vi "Get Node Reference.vi"(8 "error in":errorcluster, 11 "Item Ref in":u64 format="%.0x") -> (0 "error out":errorcluster, 2 "Base Node Type":refnum<k24>, 3 "Item Ref out":u64 format="%.0x", 4 "Base Node":refnum<k24>)   [LabVIEW 2026, in "Template Configuration.lvlib"]
uses:
  Template Configuration.lvlib
  NationalInstruments.VeriStand.SystemStorage
  NationalInstruments.VeriStand.SystemDefinitionAPI
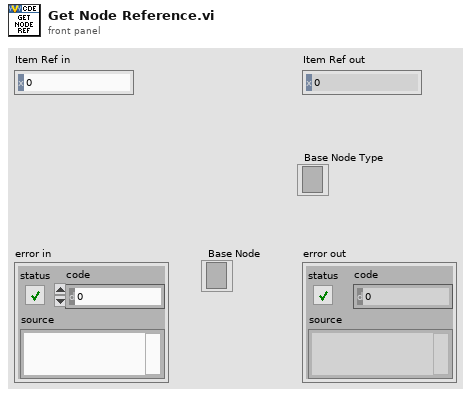
[diagram p1: front panel]
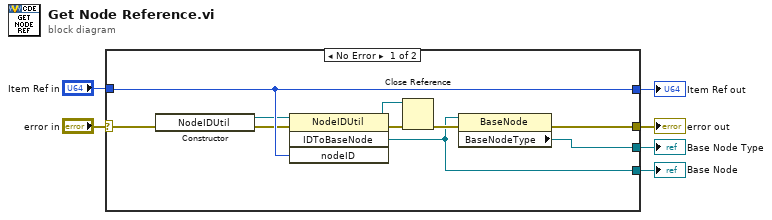
[diagram p0: block diagram]
diagram:
  n1 = case shown="No Error" "error in" {
    selector: "error in" -> [w16 w18]
    tunnel: [w15 w18] -> w5
    tunnel: [w14 _] -> w4
    tunnel: "Item Ref in" -> [w13 w17]
    tunnel: [w13 w17] -> w2
    tunnel: [w7 _] -> w1
    frame No Error {
      n2 = constructor class="NodeIDUtil"(error in=w16) -> (reference out=w8:refnum<k24>, error out=w10:errorcluster)  [unwired: 2 in, 1 out]
      n3 = invoke class="NodeIDUtil" method="IDToBaseNode"(reference=w8, error in=w10, "nodeID"=w13) -> (reference out=w9:refnum<k24>, error out=w11:errorcluster, "IDToBaseNode"=w7:refnum<k24>)  [unwired: 1 in, 1 out]
      n4 = Close Reference(reference=w9, error in (no error)=w11) -> (error out=w12:errorcluster)
      n5 = property class="BaseNode"(reference=w7, error in=w12) -> (error out=w15:errorcluster, "BaseNodeType"=w14:refnum<k24>)  [unwired: 1 out]
    }
    frame Error {
    }
  }
  "error out" <- w5
  "Base Node Type" <- w4
  "Item Ref out" <- w2
  "Base Node" <- w1
